vi "Camera Control.vi"(0 "control_camera_frames":dbl, 1 "control_saving_file_path":string, 2 "control_request":string, 5 "control_camera_exposure_time":dbl, 7 "control_camera_width":u16, 9 "control_library_reference":refnum<k24>, 11 "control_camera_reference":refnum<k24>) -> (3 "indicator_camera_status":bool, 4 "indicator_library_reference":refnum<k24>, 6 "indicator_camera_reference":refnum<k24>, 10 "Is Idle":bool, 15 "indicator_camera_buffer_index":u32)   [LabVIEW 2020]
uses:
  C:/Users/Public/Documents/Photometrics/PMQI-LabViewSamples/Examples/2018/Dependencies/PVCamNET.dll
  Public/Documents/Photometrics/PMQI-LabViewSamples/Examples/2018/Dependencies/PVCamNET.dll
panel:
  out "error out 3":errorcluster
  out "error out 2":errorcluster
  out "error out":errorcluster
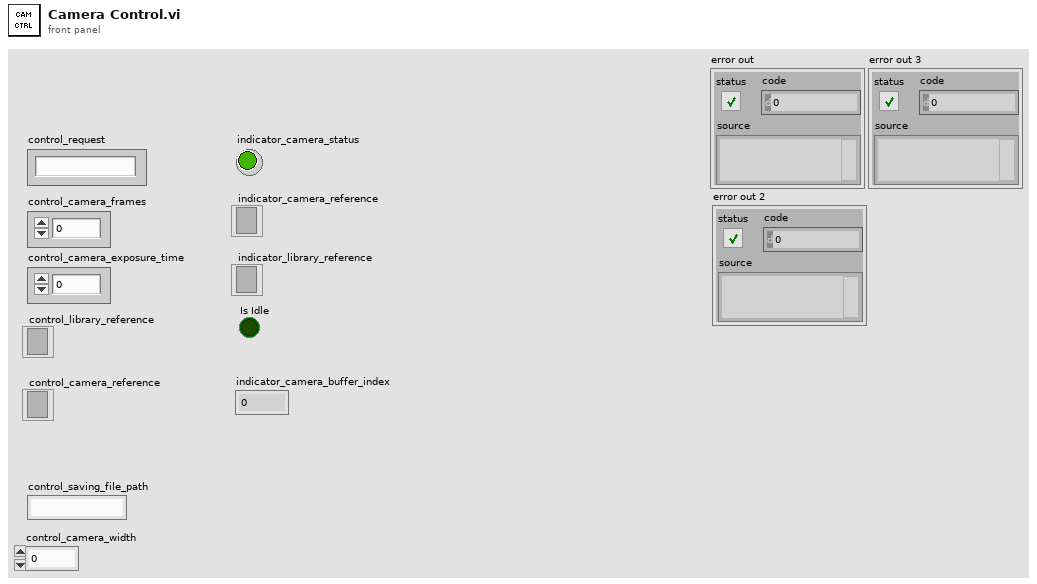
[diagram p1: front panel]
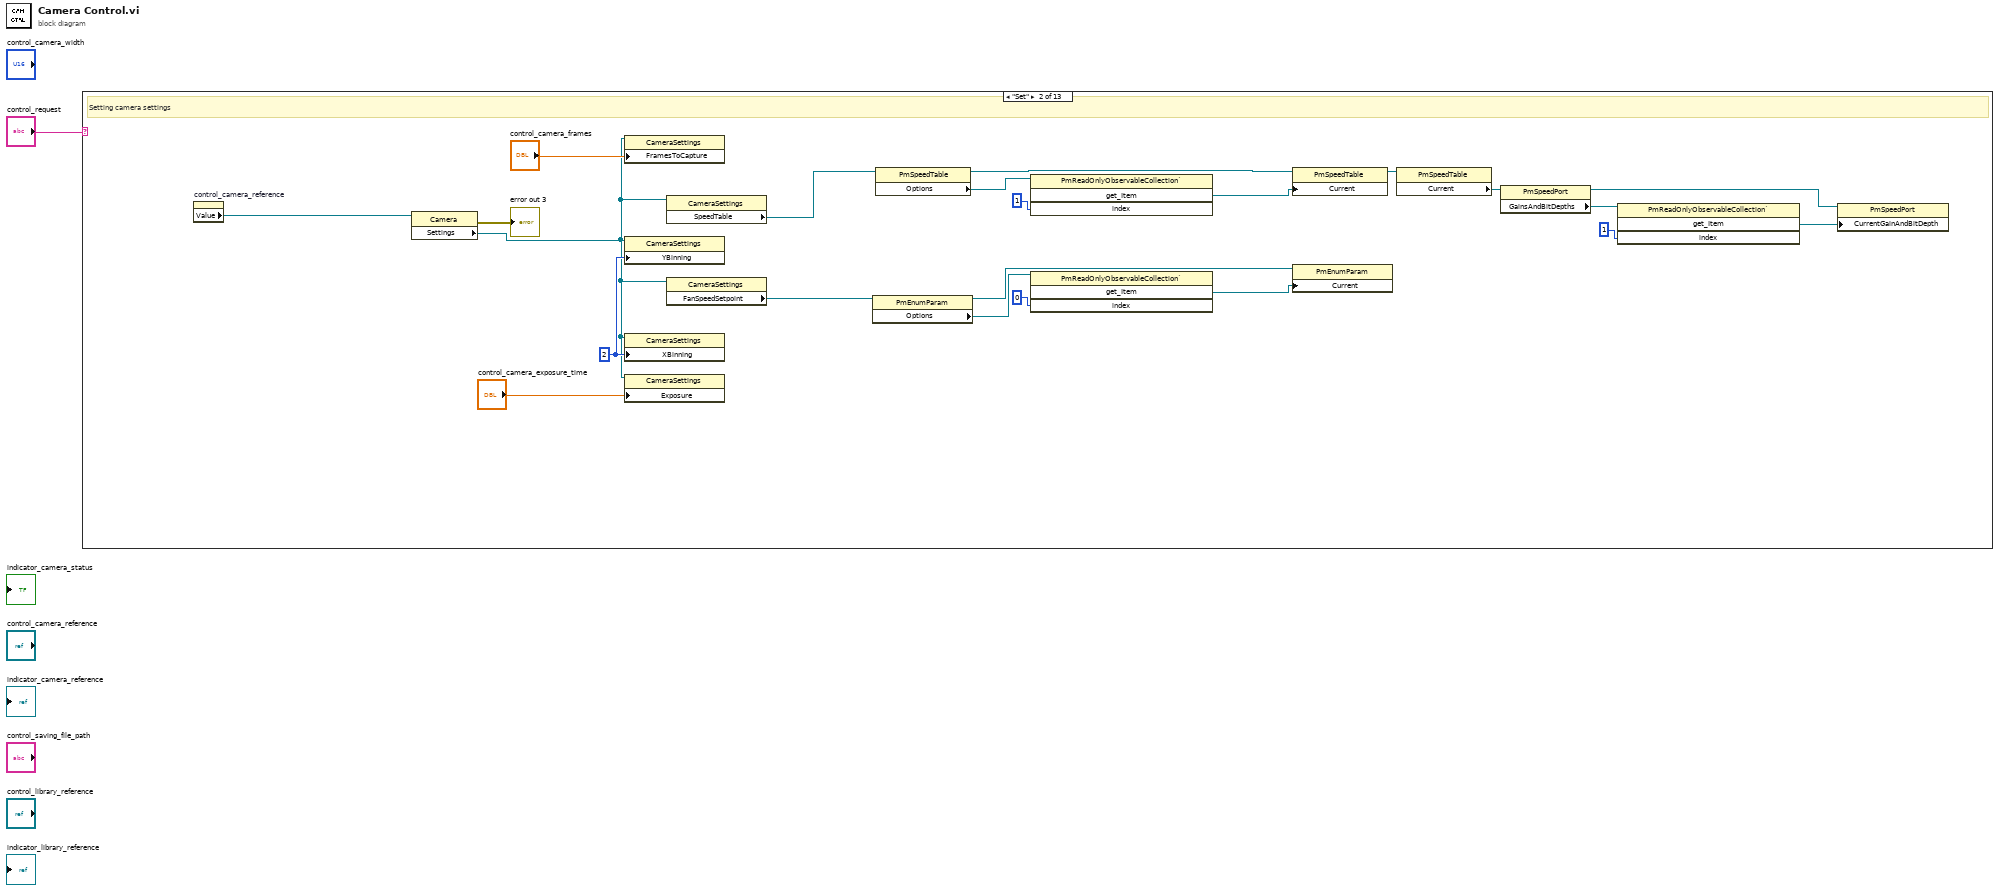
[diagram p0: block diagram]
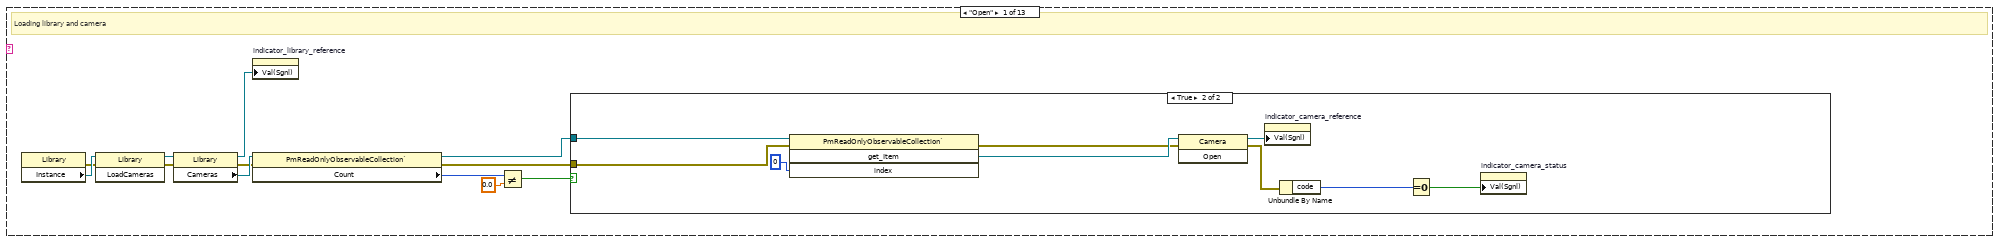
[diagram p2: hidden frame]
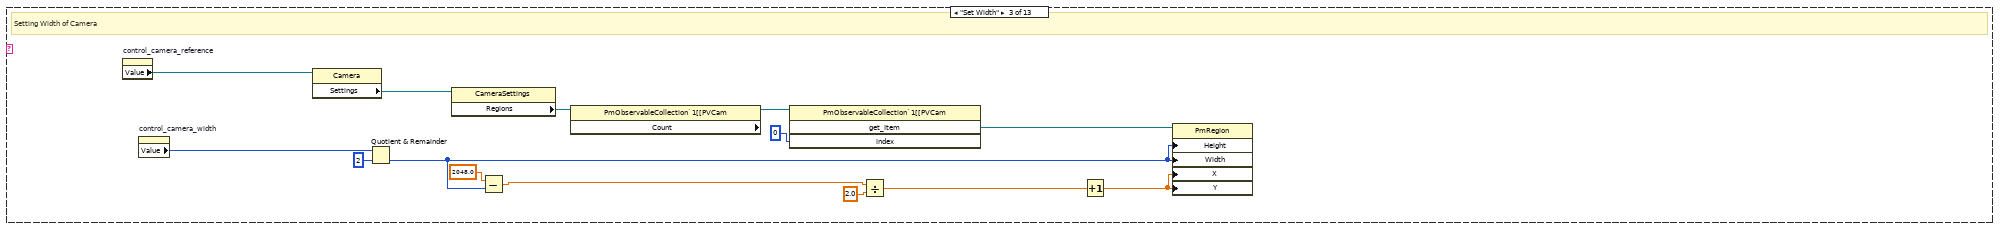
[diagram p4: hidden frame]
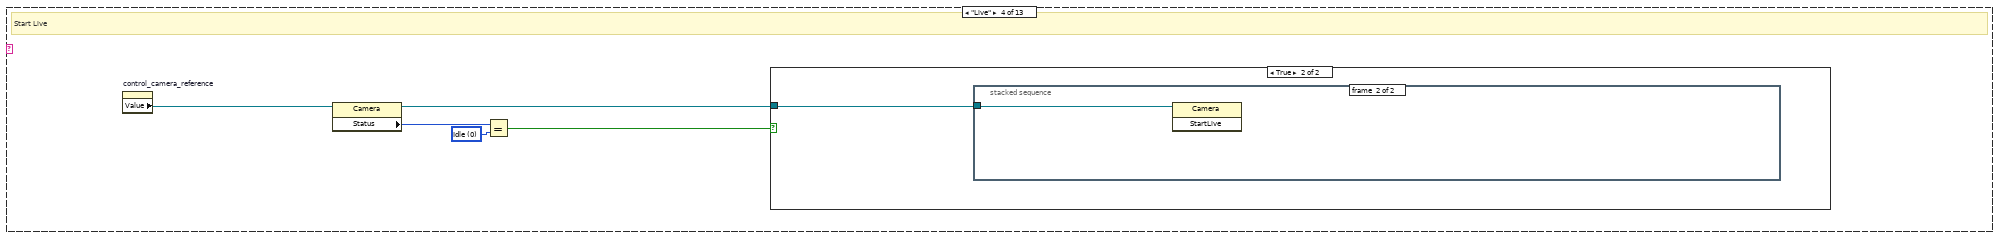
[diagram p5: hidden frame]
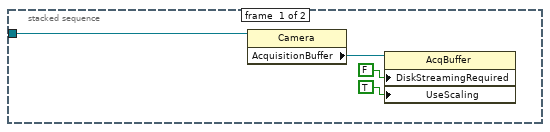
[diagram p7: hidden frame]
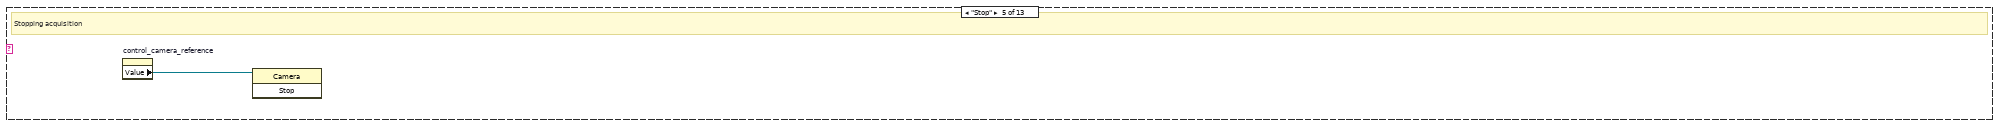
[diagram p8: hidden frame]
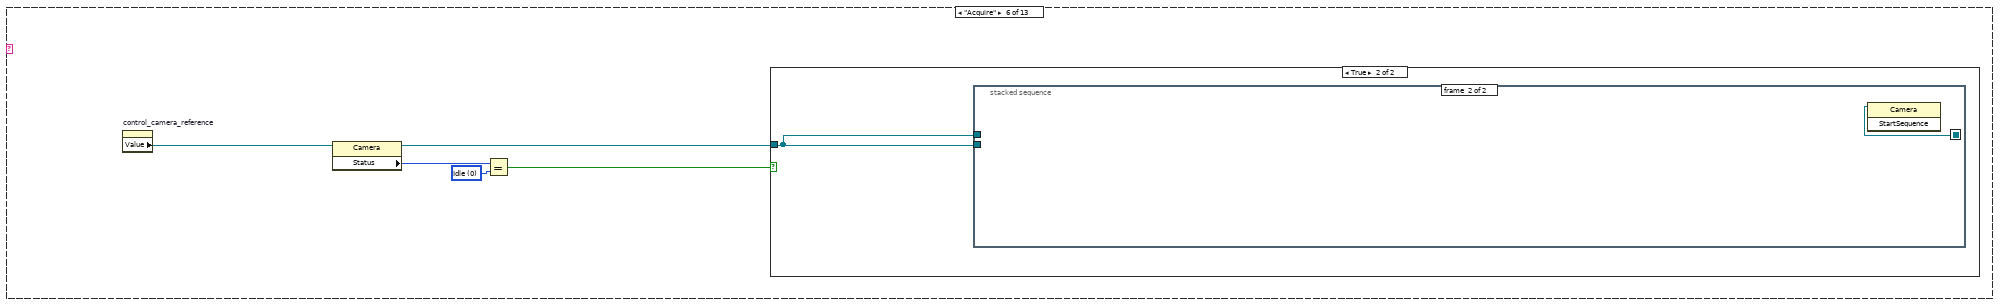
[diagram p9: hidden frame]
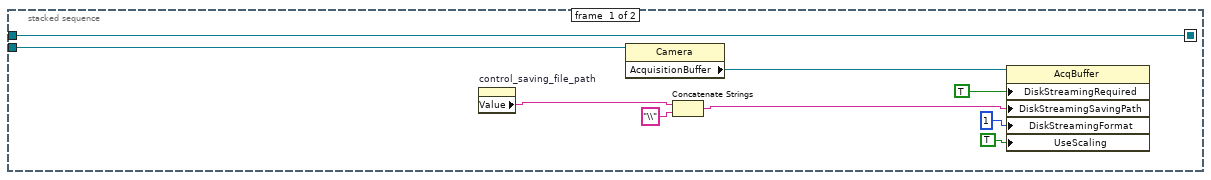
[diagram p11: hidden frame]
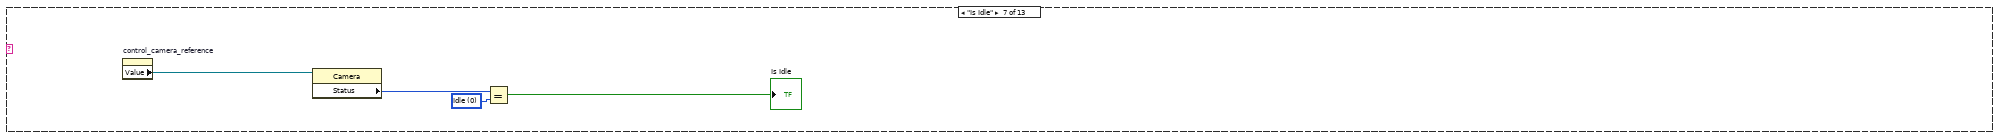
[diagram p12: hidden frame]
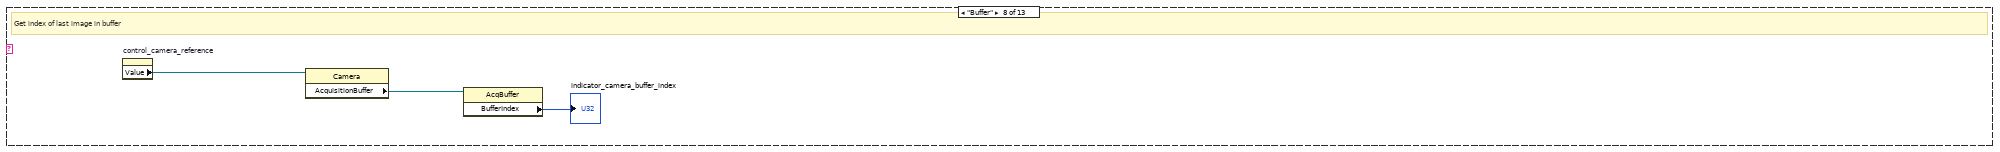
[diagram p13: hidden frame]
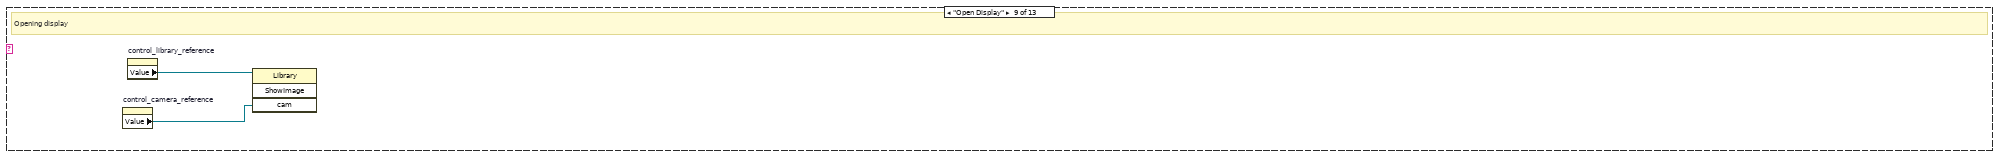
[diagram p14: hidden frame]
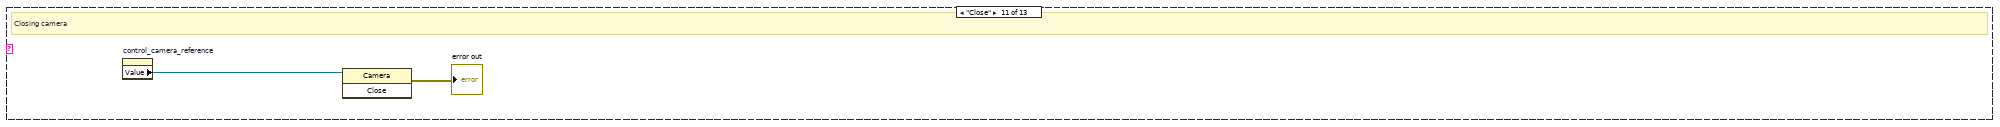
[diagram p16: hidden frame]
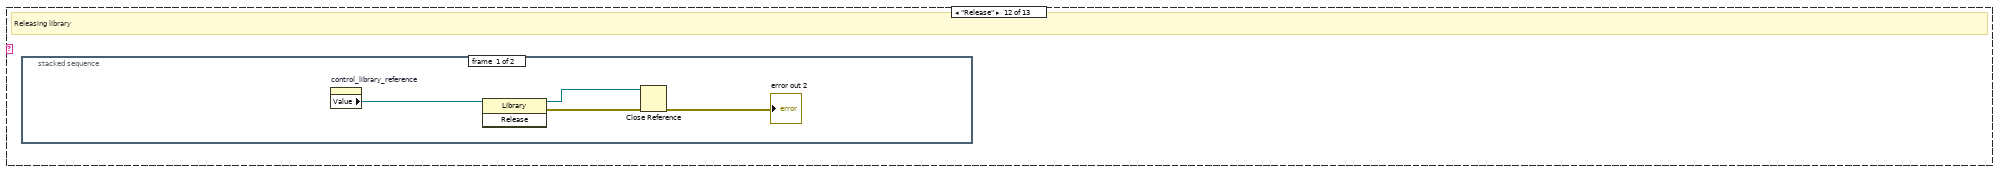
[diagram p17: hidden frame]
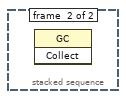
[diagram p18: hidden frame]
diagram:
  n1 = case shown="\"Set\"" "control_request" {
    frame "Open" {
      # "Loading library and camera"
      n2 = property on="Property Node" class="Library"() -> (error out=w7:errorcluster, "Instance"=w13:refnum<k24>)  [unwired: 2 in, 1 out]
      n3 = invoke class="Library" method="LoadCameras"(reference=w13, error in=w7) -> (reference out=w12:refnum<k24>, error out=w6:errorcluster)  [unwired: 1 in, 1 out]
      n4 = property class="Library"(reference=w12, error in=w6) -> (reference out=w2:refnum<k24>, error out=w5:errorcluster, "Cameras"=w11:refnum<k24>)
      n5 = property on="indicator_library_reference" class="Ref (strict)"("Val(Sgnl)"=w2) -> ()  [unwired: 2 in, 2 out]
      n6 = property class="PmReadOnlyObservableCollection`"(reference=w11, error in=w5) -> (reference out=w8:refnum<k24>, error out=w4:errorcluster, "Count"=w9:i32)
      n7 = Not Equal?(x=w9, y=0.0) -> (x != y?=w3:bool)
      n8 = case shown="True" w3 {
        tunnel: w8 -> [_ w21]
        tunnel: w4 -> [_ w20]
        frame False {
        }
        frame True {
          n9 = invoke class="PmReadOnlyObservableCollection`" method="get_Item"(reference=w21, error in=w20, "index"=0) -> (error out=w19:errorcluster, "get_Item"=w22:refnum<k24>)  [unwired: 1 in, 2 out]
          n10 = invoke class="Camera" method="Open"(reference=w22, error in=w19) -> (reference out=w17:refnum<k24>, error out=w18:errorcluster)  [unwired: 1 in, 1 out]
          n11 = property on="indicator_camera_reference" class="Ref (strict)"("Val(Sgnl)"=w17) -> ()  [unwired: 2 in, 2 out]
          n12 = Unbundle By Name(w18) -> ("code"=w15:i32)
          n13 = Equal To 0?(x=w15) -> (x = 0?=w14:bool)
          n14 = property on="indicator_camera_status" class="Bool (strict)"("Val(Sgnl)"=w14) -> ()  [unwired: 2 in, 2 out]
        }
      }
    }
    frame "Set" {
      w42 = u16 2 ("XBinning")
      # "Setting camera settings"
      n15 = property on="control_camera_reference" class="Ref (strict)"() -> ("Value"=w29:refnum<k24>)  [unwired: 2 in, 2 out]
      n16 = property class="Camera"(reference=w29) -> (error out=→"error out 3":errorcluster, "Settings"=w23:refnum<k24>)  [unwired: 1 in, 1 out]
      n17 = property class="CameraSettings"(reference=w23, "FramesToCapture"="control_camera_frames") -> ()  [unwired: 1 in, 2 out]
      n18 = property class="CameraSettings"(reference=w23, "YBinning"=w42) -> ()  [unwired: 1 in, 2 out]
      n19 = property class="CameraSettings"(reference=w23, "XBinning"=w42) -> ()  [unwired: 1 in, 2 out]
      n20 = property class="CameraSettings"(reference=w23, "Exposure"="control_camera_exposure_time") -> ()  [unwired: 1 in, 2 out]
      n21 = property class="CameraSettings"(reference=w23) -> ("SpeedTable"=w41:refnum<k24>)  [unwired: 1 in, 2 out]
      n22 = property class="CameraSettings"(reference=w23) -> ("FanSpeedSetpoint"=w28:refnum<k24>)  [unwired: 1 in, 2 out]
      n23 = property class="PmEnumParam"(reference=w28) -> (reference out=w25:refnum<k24>, "Options"=w27:refnum<k24>)  [unwired: 1 in, 1 out]
      n24 = property class="PmSpeedTable"(reference=w41) -> (reference out=w37:refnum<k24>, "Options"=w40:refnum<k24>)  [unwired: 1 in, 1 out]
      n25 = invoke class="PmReadOnlyObservableCollection`" method="get_Item"(reference=w40, "index"=1) -> ("get_Item"=w38:refnum<k24>)  [unwired: 2 in, 3 out]
      n26 = invoke class="PmReadOnlyObservableCollection`" method="get_Item"(reference=w27, "index"=0) -> ("get_Item"=w24:refnum<k24>)  [unwired: 2 in, 3 out]
      n27 = property class="PmSpeedTable"(reference=w37, "Current"=w38) -> (reference out=w36:refnum<k24>)  [unwired: 1 in, 1 out]
      n28 = property class="PmEnumParam"(reference=w25, "Current"=w24) -> ()  [unwired: 1 in, 2 out]
      n29 = property class="PmSpeedTable"(reference=w36) -> ("Current"=w35:refnum<k24>)  [unwired: 1 in, 2 out]
      n30 = property class="PmSpeedPort"(reference=w35) -> (reference out=w31:refnum<k24>, "GainsAndBitDepths"=w34:refnum<k24>)  [unwired: 1 in, 1 out]
      n31 = invoke class="PmReadOnlyObservableCollection`" method="get_Item"(reference=w34, "index"=1) -> ("get_Item"=w32:refnum<k24>)  [unwired: 2 in, 3 out]
      n32 = property class="PmSpeedPort"(reference=w31, "CurrentGainAndBitDepth"=w32) -> ()  [unwired: 1 in, 2 out]
    }
    frame "Set Width" {
      # "Setting Width of Camera"
      n33 = property on="control_camera_reference" class="Ref (strict)"() -> ("Value"=w55:refnum<k24>)  [unwired: 2 in, 2 out]
      n34 = property on="control_camera_width" class="DigNum (strict)"() -> ("Value"=w47:u16)  [unwired: 2 in, 2 out]
      n35 = property class="Camera"(reference=w55) -> ("Settings"=w58:refnum<k24>)  [unwired: 1 in, 2 out]
      n36 = Quotient & Remainder(x=w47, y=u16 2) -> (floor(x/y)=w45:u16)  [unwired: 1 out]
      n37 = property class="CameraSettings"(reference=w58) -> ("Regions"=w57:refnum<k24>)  [unwired: 1 in, 2 out]
      n38 = Subtract(x=2048.0, y=w45) -> (x-y=w51:dbl)
      n39 = property class="PmObservableCollection`1[[PVCam" props=["Count"](reference=w57) -> (reference out=w56:refnum<k24>)  [unwired: 1 in, 2 out]
      n40 = invoke class="PmObservableCollection`1[[PVCam" method="get_Item"(reference=w56, "index"=0) -> ("get_Item"=w54:refnum<k24>)  [unwired: 2 in, 3 out]
      n41 = Divide(x=w51, y=2.0) -> (x/y=w49:dbl)
      n42 = Increment(x=w49) -> (x+1=w48:dbl)
      n43 = property class="PmRegion"(reference=w54, "Height"=w45, "Width"=w45, "X"=w48, "Y"=w48) -> ()  [unwired: 1 in, 2 out]
    }
    frame "Live" {
      w61 = 0 items=["Idle", "Capturing"] ("Status")
      # "Start Live"
      n44 = property on="control_camera_reference" class="Ref (strict)"() -> ("Value"=w63:refnum<k24>)  [unwired: 2 in, 2 out]
      n45 = property class="Camera"(reference=w63) -> (reference out=w59:refnum<k24>, "Status"=w62:i32)  [unwired: 1 in, 1 out]
      n46 = Equal?(x=w62, y=w61) -> (x = y?=w60:bool)
      n47 = case shown="True" w60 {
        tunnel: w59 -> [_ w64]
        frame False {
        }
        frame True {
          n48 = stacked-sequence {
            tunnel: w64 -> [w68 w69]
            frame #0 {
              n49 = property class="Camera"(reference=w68) -> ("AcquisitionBuffer"=w67:refnum<k24>)  [unwired: 1 in, 2 out]
              n50 = property class="AcqBuffer"(reference=w67, "DiskStreamingRequired"=FALSE, "UseScaling"=TRUE) -> ()  [unwired: 1 in, 2 out]
            }
            frame #1 {
              n51 = invoke class="Camera" method="StartLive"(reference=w69) -> ()  [unwired: 2 in, 3 out]
            }
          }
        }
      }
    }
    frame "Stop" {
      # "Stopping acquisition"
      n52 = property on="control_camera_reference" class="Ref (strict)"() -> ("Value"=w70:refnum<k24>)  [unwired: 2 in, 2 out]
      n53 = invoke class="Camera" method="Stop"(reference=w70) -> ()  [unwired: 2 in, 3 out]
    }
    frame "Acquire" {
      w74 = 0 items=["Idle", "Capturing"] ("Status")
      n54 = property on="control_camera_reference" class="Ref (strict)"() -> ("Value"=w73:refnum<k24>)  [unwired: 2 in, 2 out]
      n55 = property class="Camera"(reference=w73) -> (reference out=w71:refnum<k24>, "Status"=w75:i32)  [unwired: 1 in, 1 out]
      n56 = Equal?(x=w75, y=w74) -> (x = y?=w72:bool)
      n57 = case shown="True" w72 {
        tunnel: w71 -> [_ w76]
        frame False {
        }
        frame True {
          n58 = stacked-sequence {
            seq-local: [w85 _] -> [_ w86]
            tunnel: w76 -> [w85 _]
            tunnel: w76 -> [w82 _]
            frame #0 {
              n59 = property on="control_saving_file_path" class="Str"() -> ("Value"=w79:string)  [unwired: 2 in, 2 out]
              n60 = property class="Camera"(reference=w82) -> ("AcquisitionBuffer"=w84:refnum<k24>)  [unwired: 1 in, 2 out]
              n61 = Concatenate Strings(w79, "\\" ("string")) -> (w77:string)
              n62 = property class="AcqBuffer"(reference=w84, "DiskStreamingRequired"=TRUE, "DiskStreamingSavingPath"=w77, "DiskStreamingFormat"=u32 1, "UseScaling"=TRUE) -> ()  [unwired: 1 in, 2 out]
            }
            frame #1 {
              n63 = invoke class="Camera" method="StartSequence"(reference=w86) -> ()  [unwired: 2 in, 3 out]
            }
          }
        }
      }
    }
    frame "Is Idle" {
      w89 = 0 items=["Idle", "Capturing"] ("Status")
      n64 = property on="control_camera_reference" class="Ref (strict)"() -> ("Value"=w88:refnum<k24>)  [unwired: 2 in, 2 out]
      n65 = property class="Camera"(reference=w88) -> ("Status"=w90:i32)  [unwired: 1 in, 2 out]
      n66 = Equal?(x=w90, y=w89) -> (x = y?=→"Is Idle":bool)
    }
    frame "Buffer" {
      # "Get index of last image in buffer"
      n67 = property on="control_camera_reference" class="Ref (strict)"() -> ("Value"=w93:refnum<k24>)  [unwired: 2 in, 2 out]
      n68 = property class="Camera"(reference=w93) -> ("AcquisitionBuffer"=w92:refnum<k24>)  [unwired: 1 in, 2 out]
      n69 = property class="AcqBuffer"(reference=w92) -> ("BufferIndex"=→"indicator_camera_buffer_index":u32)  [unwired: 1 in, 2 out]
    }
    frame "Open Display" {
      # "Opening display"
      n70 = property on="control_camera_reference" class="Ref (strict)"() -> ("Value"=w94:refnum<k24>)  [unwired: 2 in, 2 out]
      n71 = property on="control_library_reference" class="Ref (strict)"() -> ("Value"=w95:refnum<k24>)  [unwired: 2 in, 2 out]
      n72 = invoke class="Library" method="ShowImage"(reference=w95, "cam"=w94) -> ()  [unwired: 2 in, 4 out]
    }
    frame "Close Display" {
      # "Closing Display"
    }
    frame "Close" {
      # "Closing camera"
      n73 = property on="control_camera_reference" class="Ref (strict)"() -> ("Value"=w97:refnum<k24>)  [unwired: 2 in, 2 out]
      n74 = invoke class="Camera" method="Close"(reference=w97) -> (error out=→"error out":errorcluster)  [unwired: 2 in, 2 out]
    }
    frame "Release" {
      # "Releasing library"
      n75 = stacked-sequence {
        frame #0 {
          n76 = property on="control_library_reference" class="Ref (strict)"() -> ("Value"=w100:refnum<k24>)  [unwired: 2 in, 2 out]
          n77 = invoke class="Library" method="Release"(reference=w100) -> (reference out=w101:refnum<k24>, error out=w99:errorcluster)  [unwired: 2 in, 1 out]
          n78 = Close Reference(reference=w101, error in (no error)=w99) -> (error out=→"error out 2":errorcluster)
        }
        frame #1 {
          n79 = invoke class="GC" method="Collect"() -> ()  [unwired: 3 in, 3 out]
        }
      }
    }
    frame "Default", Default {
    }
  }
